vi "Reset State Machine.vi"(8 "error in (no error)":errorcluster, 11 "State Machine in":refnum<class "State Machine.lvclass">) -> (0 "error out":errorcluster, 3 "State Machine out":refnum<class "State Machine.lvclass">)   [LabVIEW 2018, in "State Machine.lvclass"]
uses:
  State Machine.lvclass
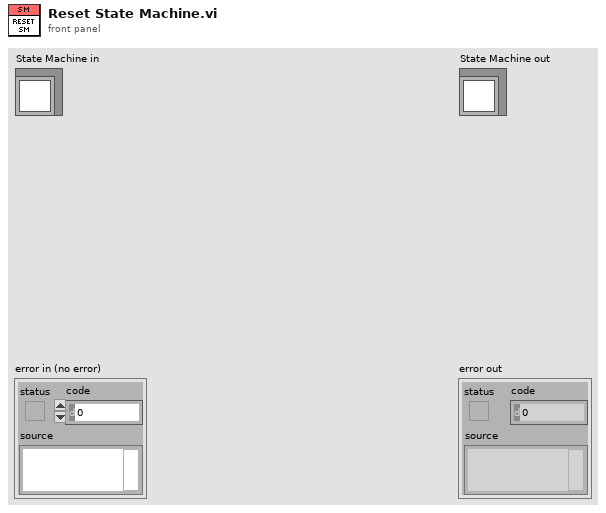
[diagram p1: front panel]
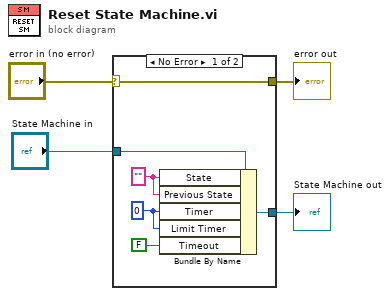
[diagram p0: block diagram]
diagram:
  n1 = case shown="No Error" "error in (no error)" {
    selector: "error in (no error)" -> [w10 w12]
    tunnel: [w10 w12] -> w2
    tunnel: [w7 w11] -> w1
    tunnel: "State Machine in" -> [w8 w11]
    frame No Error {
      w5 = "" ("State")
      w6 = u32 0
      n2 = Bundle By Name(cluster=w8, "State"=w5, "Previous State"=w5, "Timer"=w6, "Limit Timer"=w6, "Timeout"=FALSE ("timeout")) -> (w7:refnum<class "State Machine.lvclass">)
    }
    frame Error {
    }
  }
  "error out" <- w2
  "State Machine out" <- w1
